vi "Channel.OriginalName.Set.vi"(8 "error in (no error)":errorcluster, 10 "Constants.Injector.Wfm.Voltage Wfm Channel Name":string, 11 "Ref":T1 format="%.0x") -> (0 "error out":errorcluster, 3 "Ref out":T1 format="%.0x")   [LabVIEW 2015, in "Fuel Injection Addon System Explorer.lvlib"]
uses:
  Fuel Injection Addon System Explorer.lvlib
  <vilib>/NI Veristand/Custom Device API/Custom Device Item Ref.ctl
  Shared/Constants.vi
  <vilib>/NI Veristand/Custom Device API/Set Item Property (String).vi
  <vilib>/NI VeriStand/Custom Device API/Custom Device API.lvlib
  Shared/Fuel Injection Addon Shared.lvlib
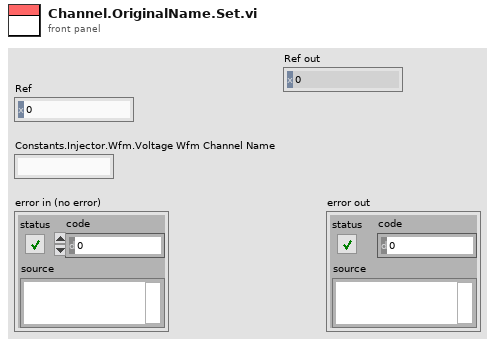
[diagram p1: front panel]
types:
  T1 = typedef "Custom Device API.lvlib/Custom Device Item Ref.ctl" = u64
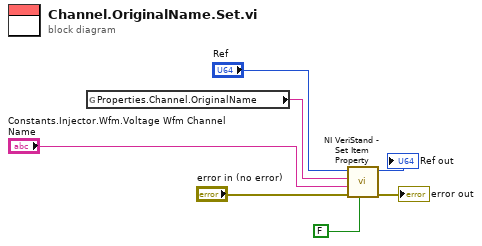
[diagram p0: block diagram]
diagram:
  n1 = global read "Constants.vi" "Properties.Channel.OriginalName"() -> (w6:string)
  n2 = call-poly <vilib>:"NI VeriStand - Set Item Property.vi"("Binary String (T)"=FALSE, "error in (no error)"="error in (no error)", "Value"="Constants.Injector.Wfm.Voltage Wfm Channel Name", "Property Name"=w6, "Item Ref in"="Ref") -> ("error out"=→"error out":errorcluster, "Item Ref out"=→"Ref out":T1)  [unwired: 4 in, 1 out]
